vi "DeCoF real query.vi"(4 "error in":errorcluster, 5 "use gsv":bool, 6 "param-name":string, 7 "Conncection ID in":T1) -> (0 "error out":errorcluster, 2 "value":dbl, 3 "Conncection ID out":T1)   [LabVIEW 2013]
uses:
  DeCoF connection.ctl
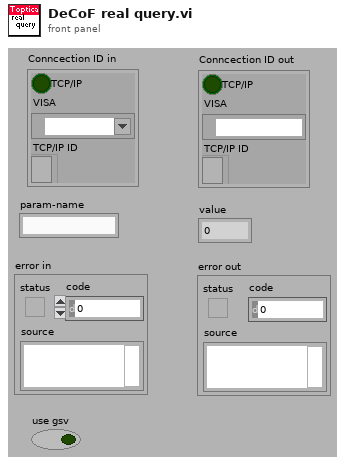
[diagram p1: front panel]
types:
  T1 = typedef "DeCoF connection.ctl" = cluster{"TCP/IP":bool, "VISA":refnum<visa-resource-name>, "TCP/IP ID":refnum<k5>}
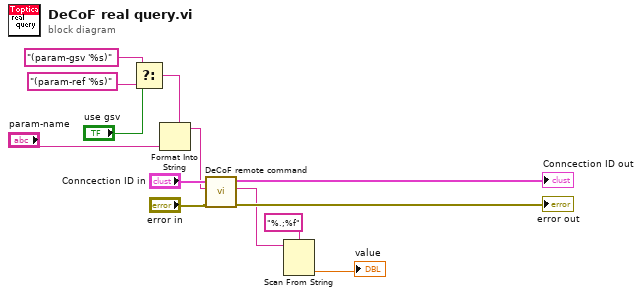
[diagram p0: block diagram]
diagram:
  n1 = Select(t="(param-gsv '%s)" ("format string"), s="use gsv", f="(param-ref '%s)" ("format string")) -> (s? t:f=w4:string)
  n2 = Format Into String(format string=w4, "param-name") -> (resulting string=w1:string)  [unwired: 2 in, 1 out]
  n3 = call "DeCoF remote command.vi"("error in (no error)"="error in", "command"=w1, "Conncection ID in"="Conncection ID in") -> ("error out"=→"error out":errorcluster, "answer string"=w9:string, "Conncection ID out"=→"Conncection ID out":T1)  [unwired: 2 in, 2 out]
  n4 = Scan From String(format string="%.;%f", input string=w9) -> (output 1=→"value":dbl)  [unwired: 3 in, 3 out]
